vi "Send acquire data request msg.vi"(1 "Message Enqueuer in":refnum<class "Message Enqueuer.lvclass">, 3 "error in (no error)":errorcluster, 4 "Message Priority (Normal)":T1=enum."Normal") -> (7 "Message Enqueuer out":refnum<class "Message Enqueuer.lvclass">, 10 "error out":errorcluster)   [LabVIEW 2015, in "Acquire data msg.lvclass"]
uses:
  Acquire data msg.lvclass
  <vilib>/ActorFramework/Message Enqueuer/Message Enqueuer.lvclass
  <vilib>/ActorFramework/Message Enqueuer/Message Priority.ctl
  <vilib>/ActorFramework/Message Enqueuer/Message Enqueuer.lvclass/Message Enqueuer.ctl
  <vilib>/ActorFramework/Message Priority Queue/Priority Enqueue.vi
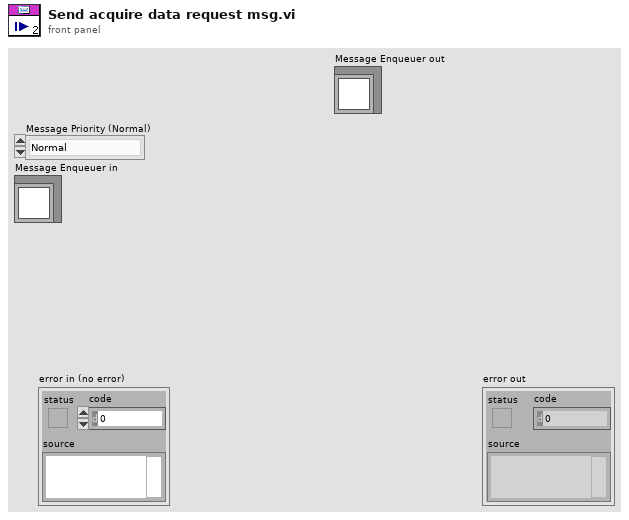
[diagram p1: front panel]
types:
  T1 = typedef "Actor Framework.lvlib/Message Enqueuer.lvclass/Message Priority.ctl" = enum16{"Low", "Normal", "High"}
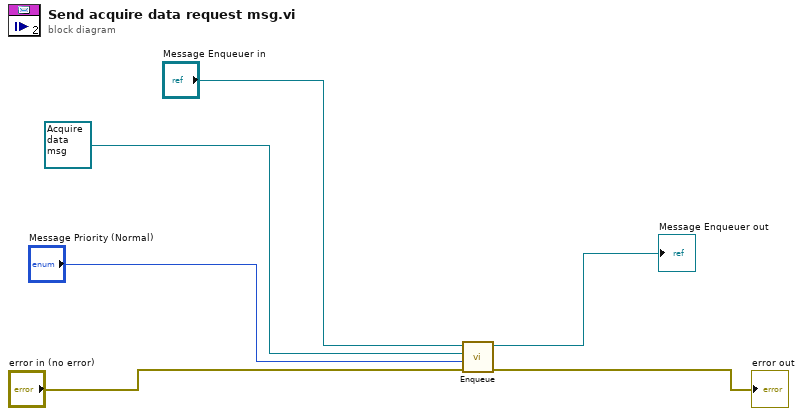
[diagram p0: block diagram]
diagram:
  n1 = call <vilib>:"Enqueue.vi"("error in (no error)"="error in (no error)", "Message Priority (Normal)"="Message Priority (Normal)", "Message"=refnum<class "Acquire data msg.lvclass"> refnum ("Acquire data msg.lvclass"), "Message Enqueuer in"="Message Enqueuer in") -> ("error out"=→"error out":errorcluster, "Message Enqueuer out"=→"Message Enqueuer out":refnum<class "Message Enqueuer.lvclass">)  [unwired: 6 in]
